vi "Equal To Core Actor.vi"(7 "Actor":refnum<class "Actor.lvclass">) -> (2 "Core Actor":bool)   [LabVIEW 2025, in "jettl.lvlib"]
uses:
  jettl.lvlib
  Actor/Actor.lvclass
  Core Actor/Core Actor.lvlib
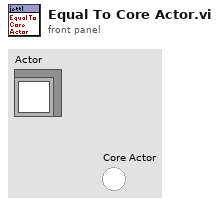
[diagram p1: front panel]
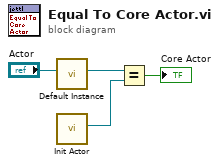
[diagram p0: block diagram]
diagram:
  n1 = call "Default Instance.vi"("Instance"="Actor") -> ("Default Instance"=w2:refnum<class "Actor.lvclass">)  [unwired: 10 in]
  n2 = call "Init Actor.vi"() -> ("Actor"=w1:refnum<class "Actor.lvclass">)  [unwired: 11 in]
  n3 = Equal?(x=w2, y=w1) -> (x = y?=→"Core Actor":bool)
